vi "(Sub VI) Parse move J.vi"(11 "data":string) -> (2 "Motion parameters":T2, 3 "Position J":T1 {"Axis 6" format="%.4f"; "Axis 5" format="%.4f"; "Axis 4" format="%.4f"; "Axis 3" format="%.4f"; "Axis 2" format="%.4f"; "Axis 1" format="%.4f"})   [LabVIEW 2022 SP3]
uses:
  <vilib>/ImagingLab/Denso Robotics Library/_Private/Controls/drl_Motion parameters.ctl
  <vilib>/ImagingLab/Denso Robotics Library/_Private/Controls/drl_Interpolation.ctl
  <vilib>/ImagingLab/Denso Robotics Library/_Private/Controls/drl_Pass motion.ctl
  <vilib>/ImagingLab/Denso Robotics Library/_Private/Controls/drl_Move option.ctl
  <vilib>/ImagingLab/Denso Robotics Library/DensoRoboticsLibrary.lvlib
  <vilib>/ImagingLab/Denso Robotics Library/_Private/Controls/drl_Variable J.ctl
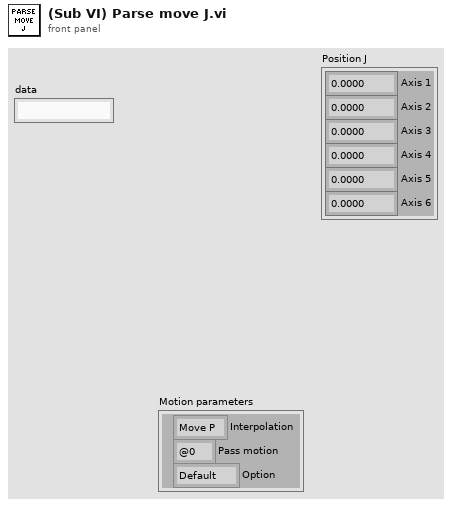
[diagram p1: front panel]
types:
  T1 = typedef "DensoRoboticsLibrary.lvlib/drl_Variable J.ctl" = cluster{"Axis 1":sgl, "Axis 2":sgl, "Axis 3":sgl, "Axis 4":sgl, "Axis 5":sgl, "Axis 6":sgl}
  T2 = typedef "DensoRoboticsLibrary.lvlib/drl_Motion parameters.ctl" = cluster{"Interpolation":T3, "Pass motion":T4, "Option":T5}
  T3 = typedef "DensoRoboticsLibrary.lvlib/drl_Interpolation.ctl" = enum16{"Move P", "Move L"}
  T4 = typedef "DensoRoboticsLibrary.lvlib/drl_Pass motion.ctl" = enum16{"@0", "@P", "@E"}
  T5 = typedef "DensoRoboticsLibrary.lvlib/drl_Move option.ctl" = enum16{"Default", "Next"}
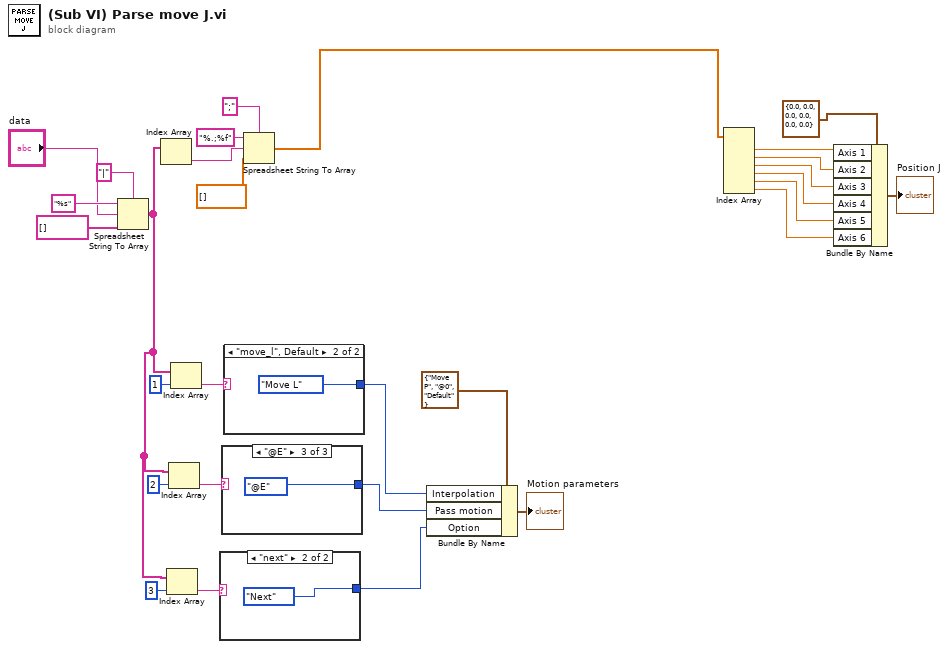
[diagram p0: block diagram]
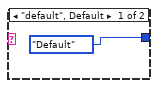
[diagram p2: hidden frame]
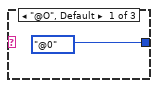
[diagram p3: hidden frame]
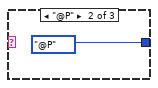
[diagram p4: hidden frame]
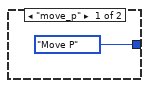
[diagram p5: hidden frame]
diagram:
  n1 = Spreadsheet String To Array(delimiter (Tab)="|", format string="%s", spreadsheet string="data", array type (2D Dbl)=string[] []) -> (array=w24:string[])
  n2 = Index Array(array=w24) -> (element=w17:string)  [unwired: 1 in]
  n3 = Index Array(array=w24, index=3) -> (element=w22:string)
  n4 = Index Array(array=w24, index=2) -> (element=w21:string)
  n5 = Index Array(array=w24, index=1) -> (element=w18:string)
  n6 = case shown="\"next\"" w22 {
    tunnel: [drl_Move_option."Default" ("Option") drl_Move_option."Next" ("Option")] -> w27
    frame "default", Default {
    }
    frame "next" {
    }
  }
  n7 = case shown="\"@E\"" w21 {
    tunnel: [drl_Pass_motion."@0" ("Pass motion") drl_Pass_motion."@P" ("Pass motion") drl_Pass_motion."@E" ("Pass motion")] -> w26
    frame "@O", Default {
    }
    frame "@P" {
    }
    frame "@E" {
    }
  }
  n8 = case shown="\"move_l\", Default" w18 {
    tunnel: [drl_Interpolation."Move P" ("Interpolation") drl_Interpolation."Move L" ("Interpolation")] -> w25
    frame "move_p" {
    }
    frame "move_l", Default {
    }
  }
  n9 = Spreadsheet String To Array(delimiter (Tab)=";", format string="%.;%f", spreadsheet string=w17, array type (2D Dbl)=dbl[] []) -> (array=w1:dbl[])
  n10 = Bundle By Name(cluster=T2 {"Interpolation"=enum."Move P", "Pass motion"=enum."@0", "Option"=enum."Default"} ("motion parameters"), "Interpolation"=w25, "Pass motion"=w26, "Option"=w27) -> (→"Motion parameters":T2)
  n11 = Index Array(array=w1) -> (element #1=w9:dbl, element #2=w8:dbl, element #3=w7:dbl, element #4=w6:dbl, element #5=w5:dbl, element #6=w4:dbl)  [unwired: 6 in]
  n12 = Bundle By Name(cluster=T1 {"Axis 1"=0.0, "Axis 2"=0.0, "Axis 3"=0.0, "Axis 4"=0.0, "Axis 5"=0.0, "Axis 6"=0.0} ("position J"), "Axis 1"=w9, "Axis 2"=w8, "Axis 3"=w7, "Axis 4"=w6, "Axis 5"=w5, "Axis 6"=w4) -> (→"Position J":T1)
